vi "readVAC.vi"(8 "error in (no error)":errorcluster) -> (0 "error out":errorcluster, 1 "medicion":dbl, 2 "Reading Result":string)   [LabVIEW 2019, in "K2002_GPIB.lvlib"]
uses:
  K2002_GPIB.lvlib
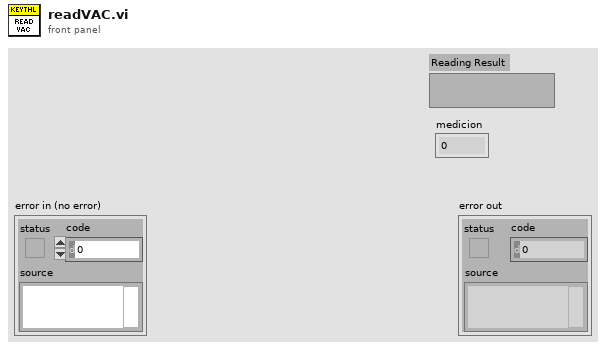
[diagram p1: front panel]
types:
  T1 = cluster{"error":bool, "code":i32, "source":string}
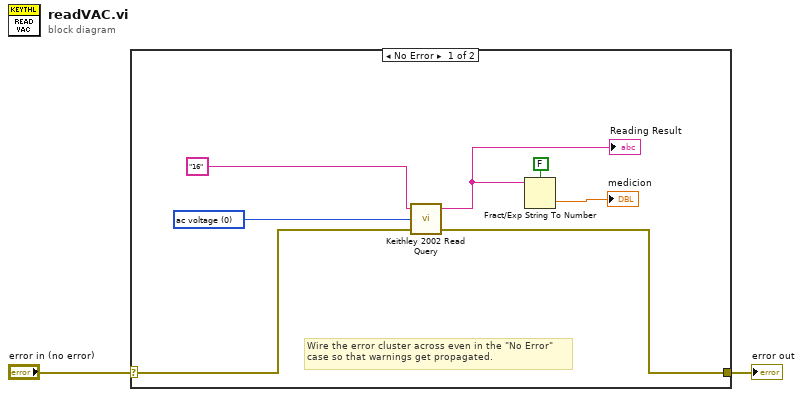
[diagram p0: block diagram]
diagram:
  n1 = case shown="No Error" "error in (no error)" {
    selector: "error in (no error)" -> [w7 w10]
    tunnel: [w3 w10] -> w1
    frame No Error {
      w9 = u16 0 items=["ac voltage", "dc voltage", "2-wire resistance", "4-wire resistance", "ac current", "dc current", "frequency", "temperature"] ("function (Vdc:1)")
      # "Wire the error cluster across even in the \"No Error\"\ncase so that warnings get propagated."
      n2 = call <instrlib>:"Keithley 2002 Read Query.vi"("error in"=w7, "function (Vdc:1)"=w9, "GPIB Address"="16") -> ("error out"=w3:T1, "Reading Result"=w6:string)  [unwired: 1 in]
      "Reading Result" <- w6
      n3 = Fract/Exp String To Number(use system decimal point (T)=FALSE, string=w6) -> (number=→"medicion":dbl)  [unwired: 2 in, 1 out]
    }
    frame Error {
    }
  }
  "error out" <- w1
